vi "iV programa 3_1.vi"() -> ()   [LabVIEW 2020]
panel:
  out "Waveform Chart":cluster{dbl, dbl}(graph)
  out "max index(es)":i32
  out "min value":dbl
  out "max value":dbl
  out "C°     F°":dbl[][](array[numeric])
  # "2.2. Genere un instrumento virtual que simule la adquisición de temperatura. Considere lo siguiente:\n• Genere 100 datos aleatorias dentro de un rango de 0 a 45.\n• Grafique los datos obtenidos.\n• Almacene los datos en un arreglo donde la primera columna deberá contener los datos originales, la segunda columna los datos representados en grados Fahrenheit.\n• La tercera columna los datos a la salida de un filtro EMA.\n• Un indicador que muestre el número máximo.\n• Otro indicador que muestre el valor mínimo."
  # "C°      F°      F° EMA"
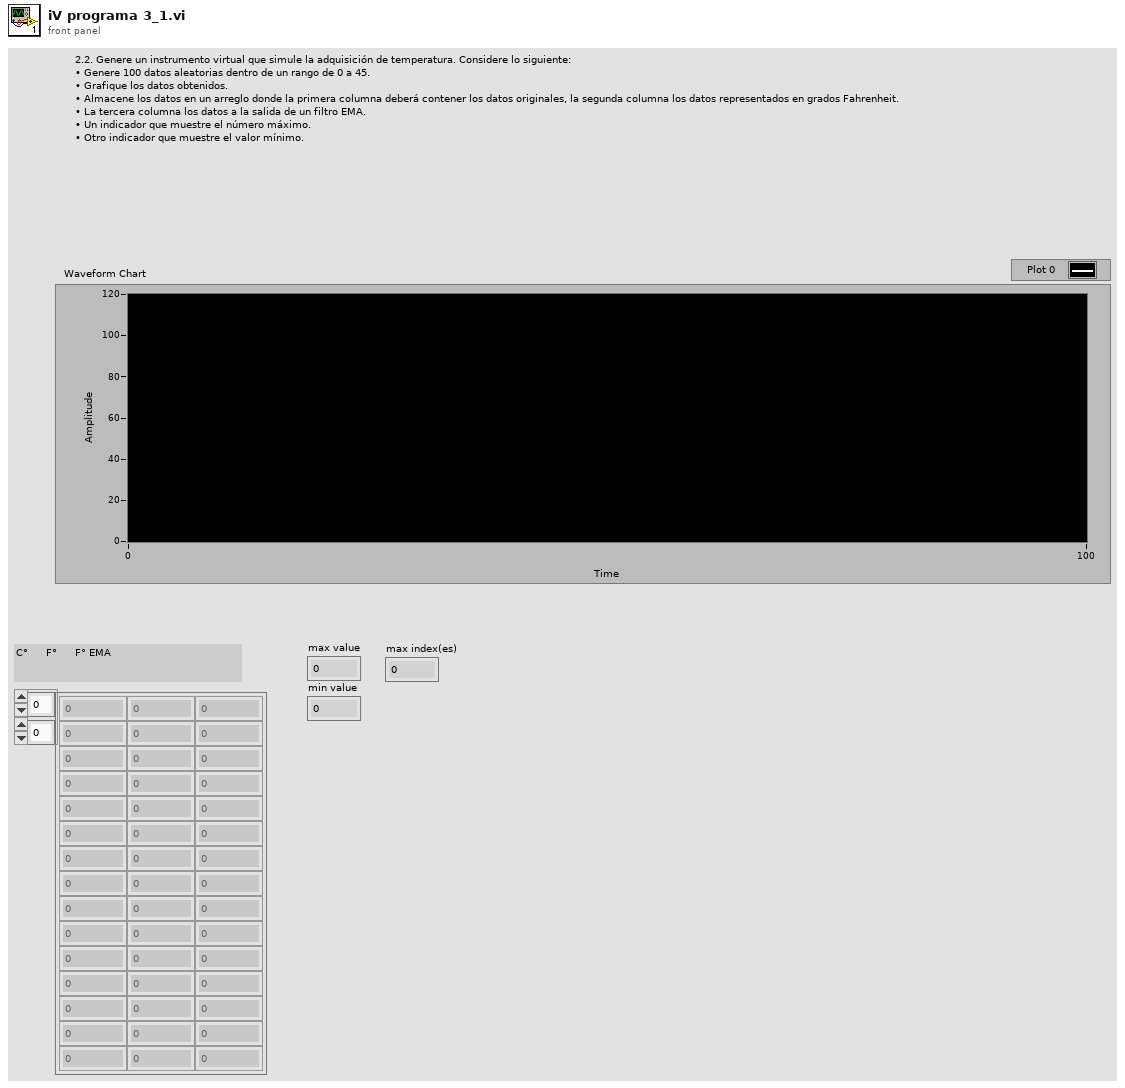
[diagram p1: front panel]
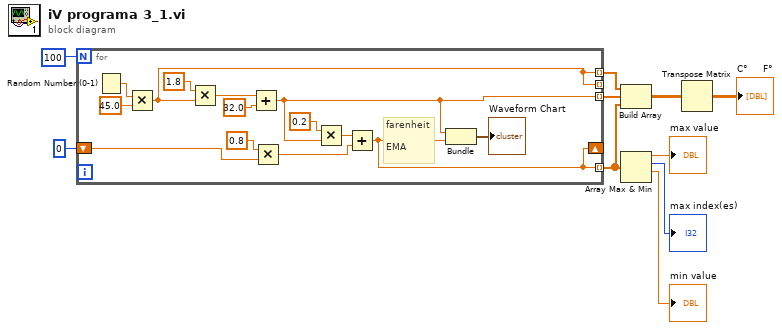
[diagram p0: block diagram]
diagram:
  n1 = for {
    N: 100 -> [_]
    tunnel: [w19] -> _ mode=indexing
    tunnel: [w12] -> w8 mode=indexing
    tunnel: [w19] -> w9 mode=indexing
    shift-right: [w13] -> _
    shift-left: 0 -> [w15]
    tunnel: [w13] -> w1 mode=indexing
    # "farenheit\n\nEMA"
    n2 = Random Number (0-1)() -> (number: 0 to 1=w24:dbl)
    n3 = Multiply(x=w24, y=45.0) -> (x*y=w19:dbl)
    n4 = Multiply(x=1.8, y=w19) -> (x*y=w21:dbl)
    n5 = Add(x=w21, y=32.0) -> (x+y=w12:dbl)
    n6 = Multiply(x=0.8, y=w15) -> (x*y=w14:dbl)
    n7 = Multiply(x=0.2, y=w12) -> (x*y=w17:dbl)
    n8 = Add(x=w17, y=w14) -> (x+y=w13:dbl)
    n9 = Bundle(w12, w13) -> (→"Waveform Chart":cluster{dbl, dbl})  [unwired: 1 in]
  }
  n10 = Build Array(w9, w8, w1) -> (w6:dbl[][])
  n11 = Array Max & Min(array=w1) -> (max value=→"max value":dbl, max index (indices)=→"max index(es)":i32, min value=→"min value":dbl)  [unwired: 1 out]
  n12 = Transpose Matrix(1:w6) -> (0:→"C°     F°":dbl[][])
